vi "array - sorted inexes - rem dup.vi"(11 "x":dbl[](array[numeric])=[1.0, 5.0, 3.0, 7.0, 0.0]) -> (1 "index array":i32[](array[numeric]), 2 "sorted array":dbl[](array[numeric]))   [LabVIEW 2015]
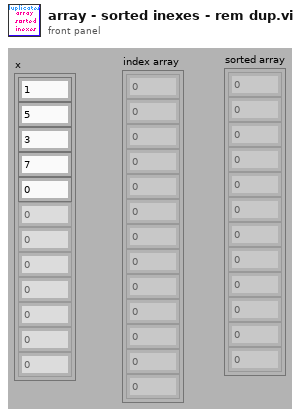
[diagram p1: front panel]
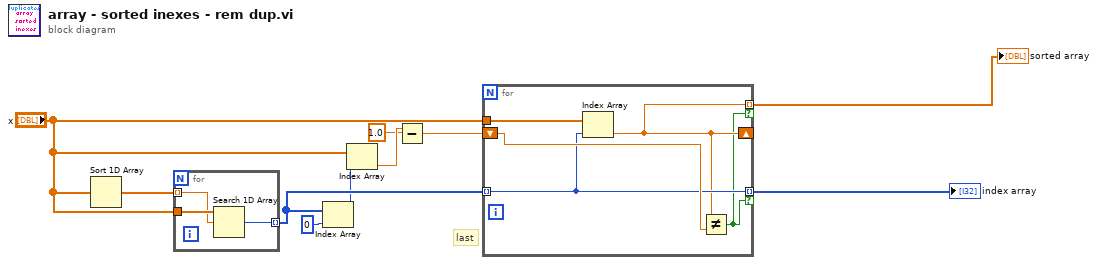
[diagram p0: block diagram]
diagram:
  # "last"
  n1 = Sort 1D Array(array="x") -> (sorted array=w10:dbl[])
  n2 = for {
    tunnel: "x" -> [w13]
    tunnel: w10 -> [w12] mode=indexing
    tunnel: [w11] -> w9 mode=indexing
    n3 = Search 1D Array(1D array=w13, element=w12) -> (index of element=w11:i32)  [unwired: 1 in]
  }
  n4 = Index Array(array=w9, index=0) -> (element=w6:i32)
  n5 = Index Array(array="x", index=w6) -> (element=w5:dbl)
  n6 = Subtract(x=w5, y=1.0) -> (x-y=w3:dbl)
  n7 = for {
    tunnel: w9 -> [w16] mode=indexing
    tunnel: "x" -> [w18]
    shift-right: [w15] -> _
    shift-left: w3 -> [w17]
    tunnel: [w16] -> w2 mode=indexing if=w14
    tunnel: [w15] -> w1 mode=indexing if=w14
    n8 = Index Array(array=w18, index=w16) -> (element=w15:dbl)
    n9 = Not Equal?(x=w15, y=w17) -> (x != y?=w14:bool)
  }
  "index array" <- w2
  "sorted array" <- w1
